vi "TL hindbrain SENSE.vi"(2 "error in":errorcluster, 3 "Power in":dbl format="%#_13g", 4 "IR Sensors":T2(array[cluster]), 5 "GPS":cluster{"X pos":i32, "Y pos":i32, "Heading":dbl}) -> (0 "error out":errorcluster, 1 "Boat Status Init":T1)   [LabVIEW 2014]
doc: "This vi calculate the distance from the boat edge to the detected object. If no object is detected the value is 0. It also determines of the boat is out of power...if so it will stop the boat."
uses:
  boatStatus.ctl
panel:
  in  "IR Max Distance":dbl=65.0
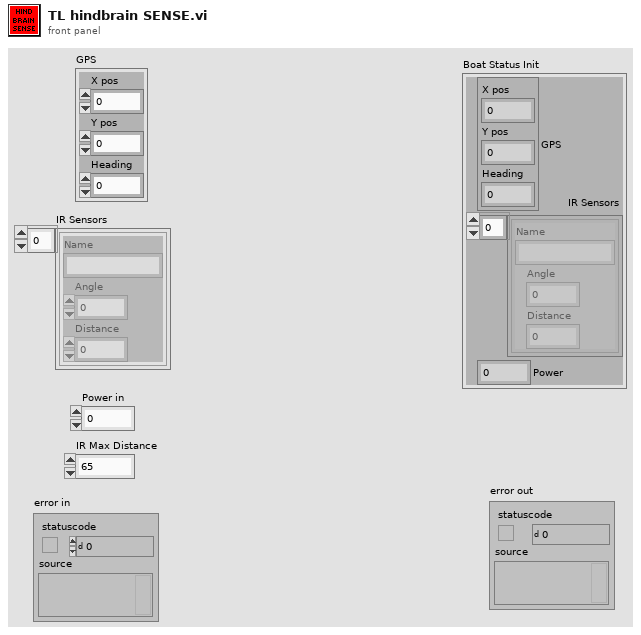
[diagram p1: front panel]
types:
  T1 = typedef "boatStatus.ctl" = cluster{"GPS":cluster{"X pos":i32, "Y pos":i32, "Heading":dbl}, "IR Sensors":cluster{"Name":string, "Angle":dbl, "Distance":dbl}[], "Power":dbl}
  T2 = cluster{"Name":string, "Angle":dbl, "Distance":dbl}[]
  T3 = cluster{"Name":string, "Angle":dbl, "Distance":dbl}
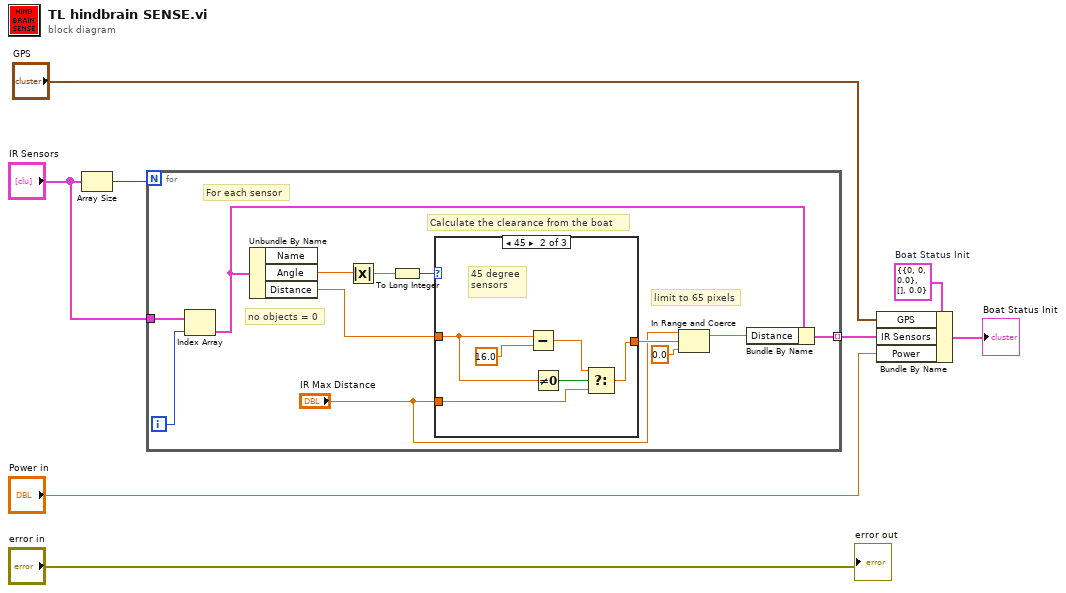
[diagram p0: block diagram]
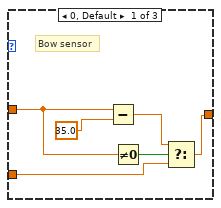
[diagram p2: hidden frame]
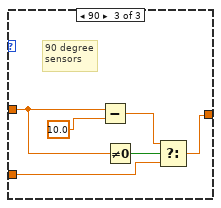
[diagram p3: hidden frame]
diagram:
  w2 = T1 {"GPS"={"X pos"=0, "Y pos"=0, "Heading"=0.0}, "IR Sensors"=[], "Power"=0.0}  # Boat Status Init
  n1 = Array Size(array="IR Sensors") -> (size(s)=w6:i32)
  n2 = for {
    N: w6 -> [_]
    tunnel: "IR Sensors" -> [w19]
    tunnel: [w14] -> w5 mode=indexing
    i -> [w18]
    # "no objects = 0"
    # "limit to 65 pixels"
    # "For each sensor"
    # "Calculate the clearance from the boat"
    n3 = Index Array(array=w19, index=w18) -> (element=w11:T3)
    n4 = Unbundle By Name(w11) -> ("Angle"=w17:dbl, "Distance"=w20:dbl)  [unwired: 1 out]
    n5 = Absolute Value(x=w17) -> (abs(x)=w16:dbl)
    n6 = To Long Integer(number=w16) -> (32bit integer=w15:i32)
    n7 = case shown="45" w15 {
      tunnel: w20 -> [w23 w29 w37]
      tunnel: [w22 w28 w34] -> w13
      tunnel: "IR Max Distance" -> [w21 w27 w33]
      frame 0, Default {
        # "Bow sensor"
        n8 = Subtract(x=w23, y=35.0) -> (x-y=w25:dbl)
        n9 = Not Equal To 0?(x=w23) -> (x != 0?=w24:bool)
        n10 = Select(t=w25, s=w24, f=w21) -> (s? t:f=w22:dbl)
      }
      frame 45 {
        # "45 degree \nsensors"
        n11 = Subtract(x=w29, y=16.0) -> (x-y=w31:dbl)
        n12 = Not Equal To 0?(x=w29) -> (x != 0?=w30:bool)
        n13 = Select(t=w31, s=w30, f=w27) -> (s? t:f=w28:dbl)
      }
      frame 90 {
        # "90 degree\nsensors"
        n14 = Subtract(x=w37, y=10.0) -> (x-y=w36:dbl)
        n15 = Not Equal To 0?(x=w37) -> (x != 0?=w38:bool)
        n16 = Select(t=w36, s=w38, f=w33) -> (s? t:f=w34:dbl)
      }
    }
    n17 = In Range and Coerce(upper limit="IR Max Distance", x=w13, lower limit=0.0) -> (coerced(x)=w10:dbl)  [unwired: 1 out]
    n18 = Bundle By Name(cluster=w11, "Distance"=w10) -> (w14:T3)
  }
  n19 = Bundle By Name(cluster=w2, "GPS"="GPS", "IR Sensors"=w5, "Power"="Power in") -> (→"Boat Status Init":T1)
  "error out" <- "error in"
